vi "Problem1.8a.vi"() -> ()   [LabVIEW 2019]
panel:
  out "Random Number Between -1 and 1":dbl
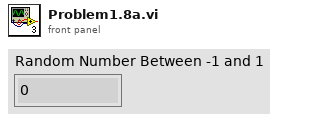
[diagram p1: front panel]
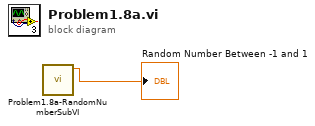
[diagram p0: block diagram]
diagram:
  n1 = call "Problem1.8a-RandomNumberSubVI.vi"() -> ("Numeric"=→"Random Number Between -1 and 1":dbl)  [unwired: 11 in]
